vi "AM Modulation Demo (Baseband-Sine) - Template.vi"() -> ()   [LabVIEW 2013]
uses:
  <vilib>/express/express analysis/Spectral/Block/exnSpectralBlock spectral measurements power poly.vi
  <vilib>/express/express analysis/Spectral/Block/exnSpectralBlock spectral measurements power DDT.vi
  <vilib>/express/express analysis/Spectral/XNode/ExpressSpectralMeasurementsBlockNode.xnode
panel:
  in  "WAV Sample Rate":dbl=44100.0 caption="dt"
  in  "Mod. Freq.":dbl=2000.0 caption="Frequency"
  in  "LPF Cut-Off":dbl=10000.0 caption="Lower Cut-Off"
  in  "AWGN (dB)":dbl(slide)=0.6 caption="Standard deviation" scale=-20.0..30.0
  out "Comparision":dynamicdata(graph)
  out "Baseband":dynamicdata(graph)
  out "AM FFT":dynamicdata(graph)
  out "AM Wave":dynamicdata(graph)
  in  "DC Offset":dbl=1.0
  in  "Carrier Amp.":dbl=1.0 caption="Amplitude"
  in  "stop":bool
  in  "Modulation Index":dbl(slide)=1.0 scale=0.0..5.0
  in  "Carrier Freq.":dbl=100000.0 caption="Frequency"
  out "After Rectifier":dynamicdata(graph)=[{"t0"=timestamp(0 s since 1904-01-01), "dt"=10.0, "Y"=array[50000 elements], "attributes"=variant("NI_ChannelName"=variant(string "Sine (Power Spectrum)"), "NI_ExpIsRelativeTime"=variant(bool TRUE), "NI_ExpStartTimeStamp"=variant(timestamp timestamp(3635665779.2842293 s since 1904-01-01)), "NI_ExpTimeStamp"=variant(timestamp timestamp(3635665779.2842293 s since 1904-01-01)), "NI_ExpXDimension"=variant(string "f"), "NI_OriginalChannelName"=variant(string "Sine"))}]
  # "Amplitude Modulation"
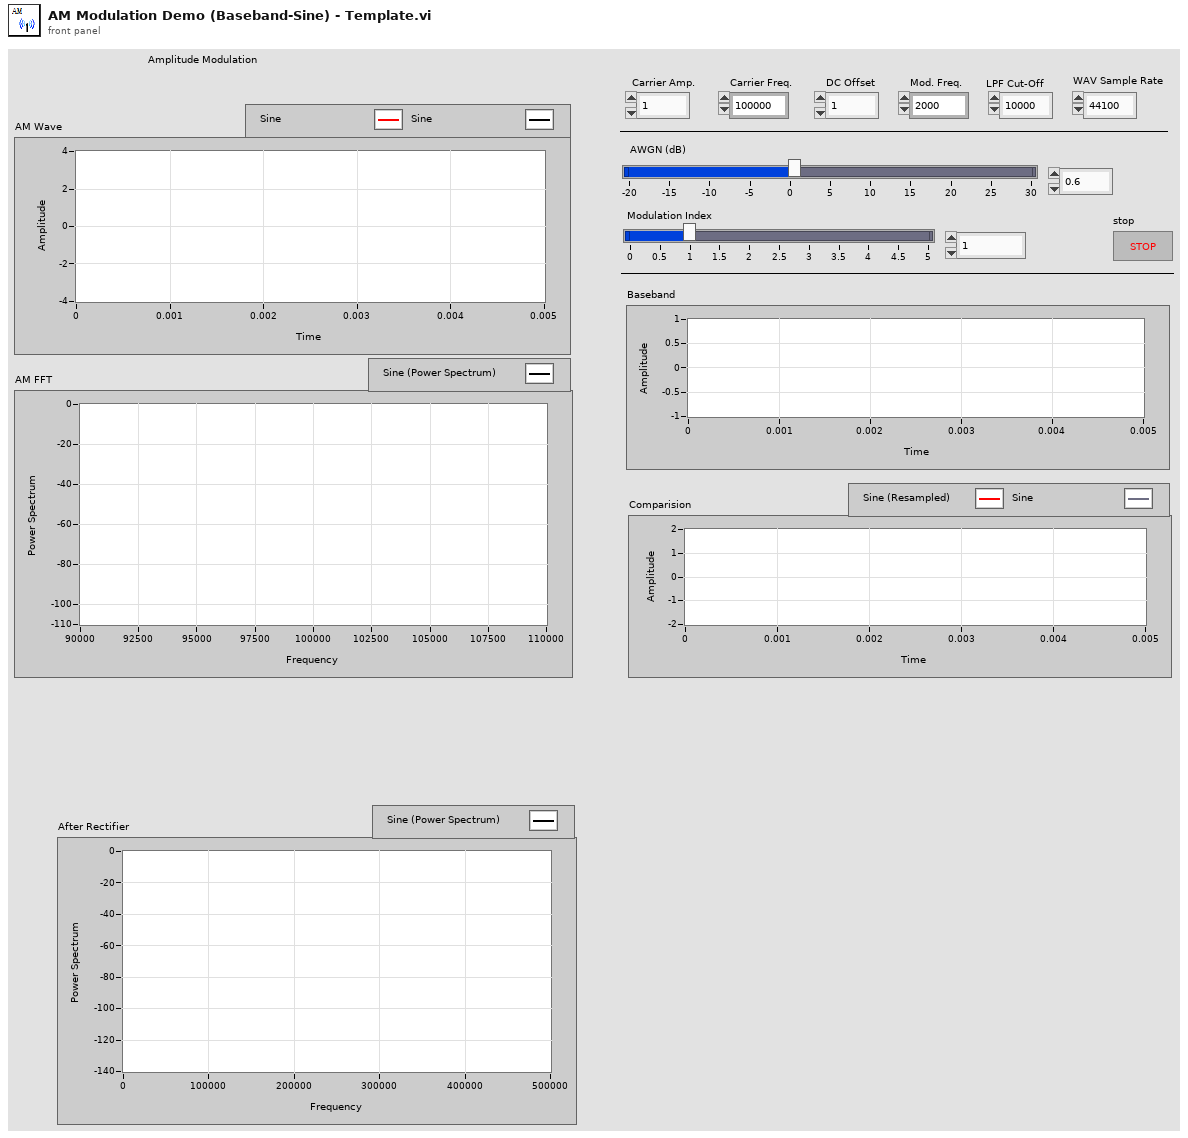
[diagram p1: front panel]
types:
  T1 = cluster{"averaging mode":u16, "weighting mode":u16, "number of averages":u32}
  T2 = cluster{"dB On (F)":bool, "unwrap phase (F)":bool, "convert to degree (F)":bool}
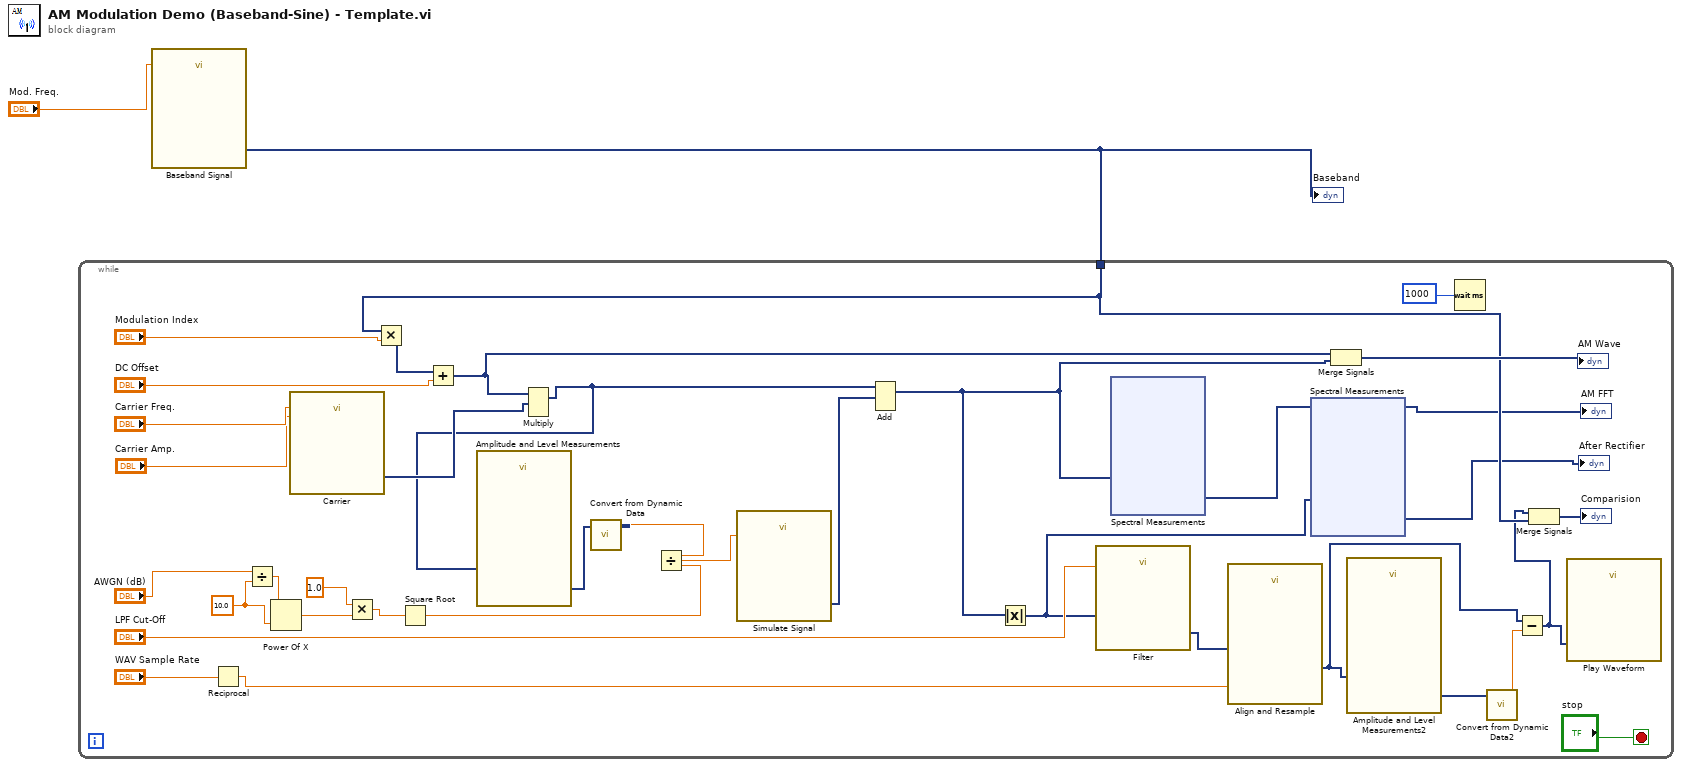
[diagram p0: block diagram]
diagram:
  n1 = call "Baseband Signal"("Frequency"="Mod. Freq.") -> ("Sine"=w1:dynamicdata)  [unwired: 13 in, 1 out]
  "Baseband" <- w1
  n2 = while {
    tunnel: w1 -> [w14]
    stop <- "stop" stop-if-true
    w10 = 10.0
    n3 = Reciprocal(x="WAV Sample Rate") -> (1/x=w18:dbl)
    n4 = Divide(x="AWGN (dB)", y=w10) -> (x/y=w11:dbl)
    n5 = Power Of X(1:w10, 2:w11) -> (0:w9:dbl)
    n6 = call "Carrier"("Frequency"="Carrier Freq.", "Amplitude"="Carrier Amp.") -> ("Sine"=w32:dynamicdata)  [unwired: 12 in, 1 out]
    n7 = Multiply(x=1.0, y=w9) -> (x*y=w25:dbl)
    n8 = Multiply(x=w14, y="Modulation Index") -> (x*y=w36:dynamicdata)
    n9 = Square Root(x=w25) -> (sqrt(x)=w23:dbl)
    n10 = Add(x=w36, y="DC Offset") -> (x+y=w30:dynamicdata)
    n11 = Multiply(1:w32, 2:w30) -> (0:w22:dynamicdata)  [unwired: 1 in, 1 out]
    n12 = call "Amplitude and Level Measurements"("Signals"=w22) -> ("RMS"=w29:dynamicdata)  [unwired: 13 in, 1 out]
    n13 = call "Convert from Dynamic Data"("Dynamic Data Type"=w29) -> ("Scalar"=w24:dbl)  [unwired: 3 in]
    n14 = Divide(x=w24, y=w23) -> (x/y=w8:dbl)
    n15 = call "Simulate Signal"("Standard deviation"=w8) -> ("DC with Gaussian Noise"=w21:dynamicdata)  [unwired: 13 in, 1 out]
    n16 = Add(1:w21, 2:w22) -> (0:w19:dynamicdata)  [unwired: 1 in, 1 out]
    n17 = Absolute Value(x=w19) -> (abs(x)=w4:dynamicdata)
    n18 = call "Filter"("Lower Cut-Off"="LPF Cut-Off", "Signal"=w4) -> ("Filtered Signal"=w17:dynamicdata)  [unwired: 8 in, 1 out]
    n19 = xnode "Spectral Measurements"("Signals"=w19) -> ("Power Spectrum"=→"AM FFT":dynamicdata)  [unwired: 1 in, 1 out]
    n20 = call "Align and Resample"("dt"=w18, "Signals"=w17) -> ("Resampled Signals"=w5:dynamicdata)  [unwired: 7 in, 2 out]
    n21 = xnode "Spectral Measurements"("Signals"=w4) -> ("Power Spectrum"=→"After Rectifier":dynamicdata)  [unwired: 1 in, 1 out]
    n22 = Merge Signals(w30, w19) -> (→"AM Wave":dynamicdata)
    n23 = call "Amplitude and Level Measurements2"("Signals"=w5) -> ("Mean (DC)"=w6:dynamicdata)  [unwired: 13 in, 1 out]
    n24 = Wait (ms)(milliseconds to wait=1000) -> ()  [unwired: 1 out]
    n25 = call "Convert from Dynamic Data2"("Dynamic Data Type"=w6) -> ("Scalar"=w13:dbl)  [unwired: 3 in]
    n26 = Subtract(x=w5, y=w13) -> (x-y=w7:dynamicdata)
    n27 = Merge Signals(w7, w14) -> (→"Comparision":dynamicdata)
    n28 = call "Play Waveform"("Data"=w7) -> ()  [unwired: 18 in, 1 out]
  }
